vi "SwerveDrive2.0.vi"(6 "Right Trigger":dbl, 8 "RCW":dbl(slide) scale=-1.0..1.0, 9 "STR":dbl(slide) scale=-1.0..1.0, 10 "FWD":dbl(slide) scale=-1.0..1.0, 11 "Gyro":dbl=-0.03423117662966245) -> ()   [LabVIEW 2023]
uses:
  <vilib>/Rock Robotics/WPI/ThirdParty/ADI/ADIS16470/Typedef/ADIS16470 Data.ctl
  <vilib>/Rock Robotics/WPI/ThirdParty/REV Robotics/REVLib/Typedef/Spark MAX Control Type.ctl
  <vilib>/addons/control/pid/NI_PID_pid.lvlib
  <vilib>/addons/control/pid/pid.llb/PID (DBL).vi
panel:
  in  "Do X Pattern":bool=TRUE
  in  "W4 PID":T1={"proportional gain (Kc)"=0.2, "integral time (Ti, min)"=0.0, "derivative time (Td, min)"=0.0}
  in  "W1 PID":T1={"proportional gain (Kc)"=0.2, "integral time (Ti, min)"=0.0, "derivative time (Td, min)"=0.0}
  in  "W2 PID":T1={"proportional gain (Kc)"=0.2, "integral time (Ti, min)"=0.0, "derivative time (Td, min)"=0.0}
  in  "W3 PID":T1={"proportional gain (Kc)"=0.2, "integral time (Ti, min)"=0.0, "derivative time (Td, min)"=0.0}
  out "ADIS16470 Value":T2
  out "W2 Encoder":dbl
  out "W1 Encoder":dbl
  out "WA 4":dbl=135.0
  out "WA 3":dbl=225.0
  out "WA 2":dbl=315.0
  out "WA 1":dbl=45.0
  out "WS 4":dbl
  out "WS 3":dbl
  out "WS 2":dbl
  out "WS 1":dbl
  out "W4 Encoder":dbl
  out "W3 Encoder":dbl
  # "0.2\n0\n0\nfor all"
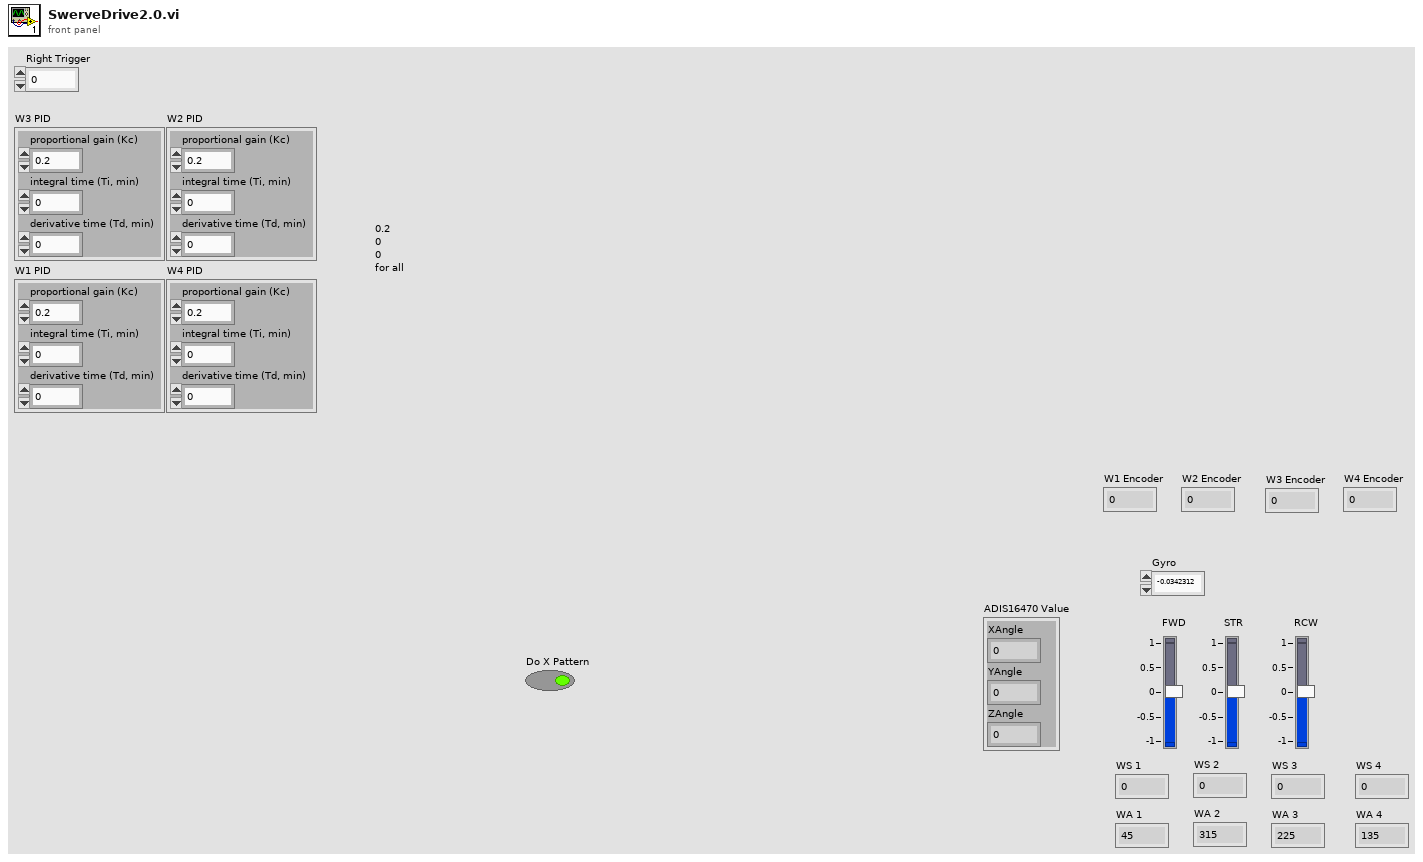
[diagram p1: front panel]
types:
  T1 = cluster{"proportional gain (Kc)":dbl, "integral time (Ti, min)":dbl, "derivative time (Td, min)":dbl}
  T2 = typedef "ADIS16470 Data.ctl" = cluster{"XAngle":dbl, "YAngle":dbl, "ZAngle":dbl}
  T3 = typedef "WPI_JoystickDevRef.ctl" = cluster{"Device":T4}
  T4 = typedef "WPI_JoystickDeviceEnum.ctl" = enum16{"USB 0", "USB 1", "USB 2", "USB 3", "USB 4", "USB 5"}
  T5 = typedef "ADIS16470 Device Reference.ctl" = cluster{"DevStatus":errorcluster, "Hardware Config":T6, "Calibration Complete":refnum<notifier>, "Status Reference":refnum<data-value>, "Data Reference":refnum<data-value>, "Sychronous Process VI":T10, "Cmd FIFO":refnum<k33>, "Source":T11, "Data FIFO":refnum<k33>, "Calibration Time (ms)":u32, "Data Reference":refnum<data-value>}
  T6 = typedef "ADIS16470 Hardware Configuration.ctl" = cluster{"SPI Clock Rate (Hz)":dbl, "IMU SPI Mode (3)":T7, "IMU Reset Pin":T8, "IMU SPI Bus":T9, "IMU Data Ready Pin":T8, "Stall Config":cluster{"Pow2BytesPerRead":u8, "StallTicks":u16, "CsToSclkTicks":u8}}
  T7 = typedef "WPI_SPIMode.ctl" = enum16{"Mode 0 (Clk Idle Low,Sample on Leading)", "Mode 1 (Clk Idle Low,Sample on Trailing)", "Mode 2 (Clk Idle High,Sample on Leading)", "Mode 3 (Clk Idle High,Sample on Trailing)"}
  T8 = typedef "FPGA_DIOChannel.ctl" = enum8{"DIO 0", "DIO 1", "DIO 2", "DIO 3", "DIO 4", "DIO 5", "DIO 6", "DIO 7", "DIO 8", "DIO 9", "DIO MXP 0", "DIO MXP 1", "DIO MXP 2", "DIO MXP 3", "DIO MXP 4", "DIO MXP 5", "DIO MXP 6", "DIO MXP 7", "DIO MXP 8", "DIO MXP 9", "DIO MXP 10", "DIO MXP 11", "DIO MXP 12", "DIO MXP 13", "DIO MXP 14", "DIO MXP 15", "SPI Port CS1", "SPI Port CS2", "SPI Port CS3", "SPI Port MISO", "SPI Port MOSI", "Invalid"}
  T9 = typedef "spi_bus.ctl" = enum16{"SPI On-Board, CS0", "SPI On-Board, CS1", "SPI On-Board, CS2", "SPI On-Board, CS3", "SPI MXP", "Invalid"}
  T10 = typedef "ADIS16470 Process.ctl" = refnum<vi>
  T11 = typedef "FPGA_CounterEncoderSourceConvertionLVSourceType.ctl" = cluster{"DevStatus":errorcluster, "AnalogTriggerMode?":bool, "DigitalMode":cluster{"DIO Channel":T12}, "AnalogTriggerMode":cluster{"AnalogTriggerIndex":T13, "OutputType":T14}}
  T12 = typedef "FPGA_DIODigitalSourceChannel.ctl" = enum8{"DIO 0", "DIO 1", "DIO 2", "DIO 3", "DIO 4", "DIO 5", "DIO 6", "DIO 7", "DIO 8", "DIO 9", "DIO MXP 0", "DIO MXP 1", "DIO MXP 2", "DIO MXP 3", "DIO MXP 4", "DIO MXP 5", "DIO MXP 6", "DIO MXP 7", "DIO MXP 8", "DIO MXP 9", "DIO MXP 10", "DIO MXP 11", "DIO MXP 12", "DIO MXP 13", "DIO MXP 14", "DIO MXP 15", "SPI Port CS1", "SPI Port CS2", "SPI Port CS3", "SPI Port MISO", "SPI Port MOSI", "Disabled"}
  T13 = typedef "FPGA_AnalogTriggerIndex.ctl" = enum8{"Trig 0", "Trig 1", "Trig 2", "Trig 3", "Trig 4", "Trig 5", "Trig 6", "Trig 7", "Invalid"}
  T14 = typedef "FPGA_AnalogTriggerOutType.ctl" = enum16{"InWindow", "TriggerState", "Rising", "Falling"}
  T15 = typedef "WPI_MotorControlDeviceRef.ctl" = cluster{"DeviceStatus":errorcluster, "Type":T16, "PWM":cluster{"PWM Channel":T17, "DeadBand":T18}, "CAN":cluster{"Device Number":u8, "SetOutput VI Ref":variant, "GetOutput VI Ref":variant, "Enable VI Ref":variant, "Disable VI Ref":variant, "Data":variant}, "Invert":bool, "DIO PWM":cluster{"PWM \"Enable\" Channel":T17, "DIOChannel":T8, "PWM Rate":dbl}}
  T16 = typedef "WPI_MotorControlType.ctl" = enum16{"PWM", "CAN", "DIO PWM"}
  T17 = typedef "FPGA_DIOPWMChannel.ctl" = enum8{"PWM 0", "PWM 1", "PWM 2", "PWM 3", "PWM 4", "PWM 5", "PWM 6", "PWM 7", "PWM 8", "PWM 9", "PWM MXP 0", "PWM MXP 1", "PWM MXP 2", "PWM MXP 3", "PWM MXP 4", "PWM MXP 5", "PWM MXP 6", "PWM MXP 7", "PWM MXP 8", "PWM MXP 9", "Invalid"}
  T18 = typedef "WPI_PWMDeadband.ctl" = cluster{"Name":string, "maxPositivePwm":i32, "minPositivePwm":i32, "centerPwm":i32, "maxNegativePwm":i32, "minNegativePwm":i32, "angularRange":u16}
  T19 = typedef "Spark MAX Control Type.ctl" = enum16{"Percent VBus", "Voltage", "Velocity", "Position", "Smart Motion", "Current", "Smart Velocity"}
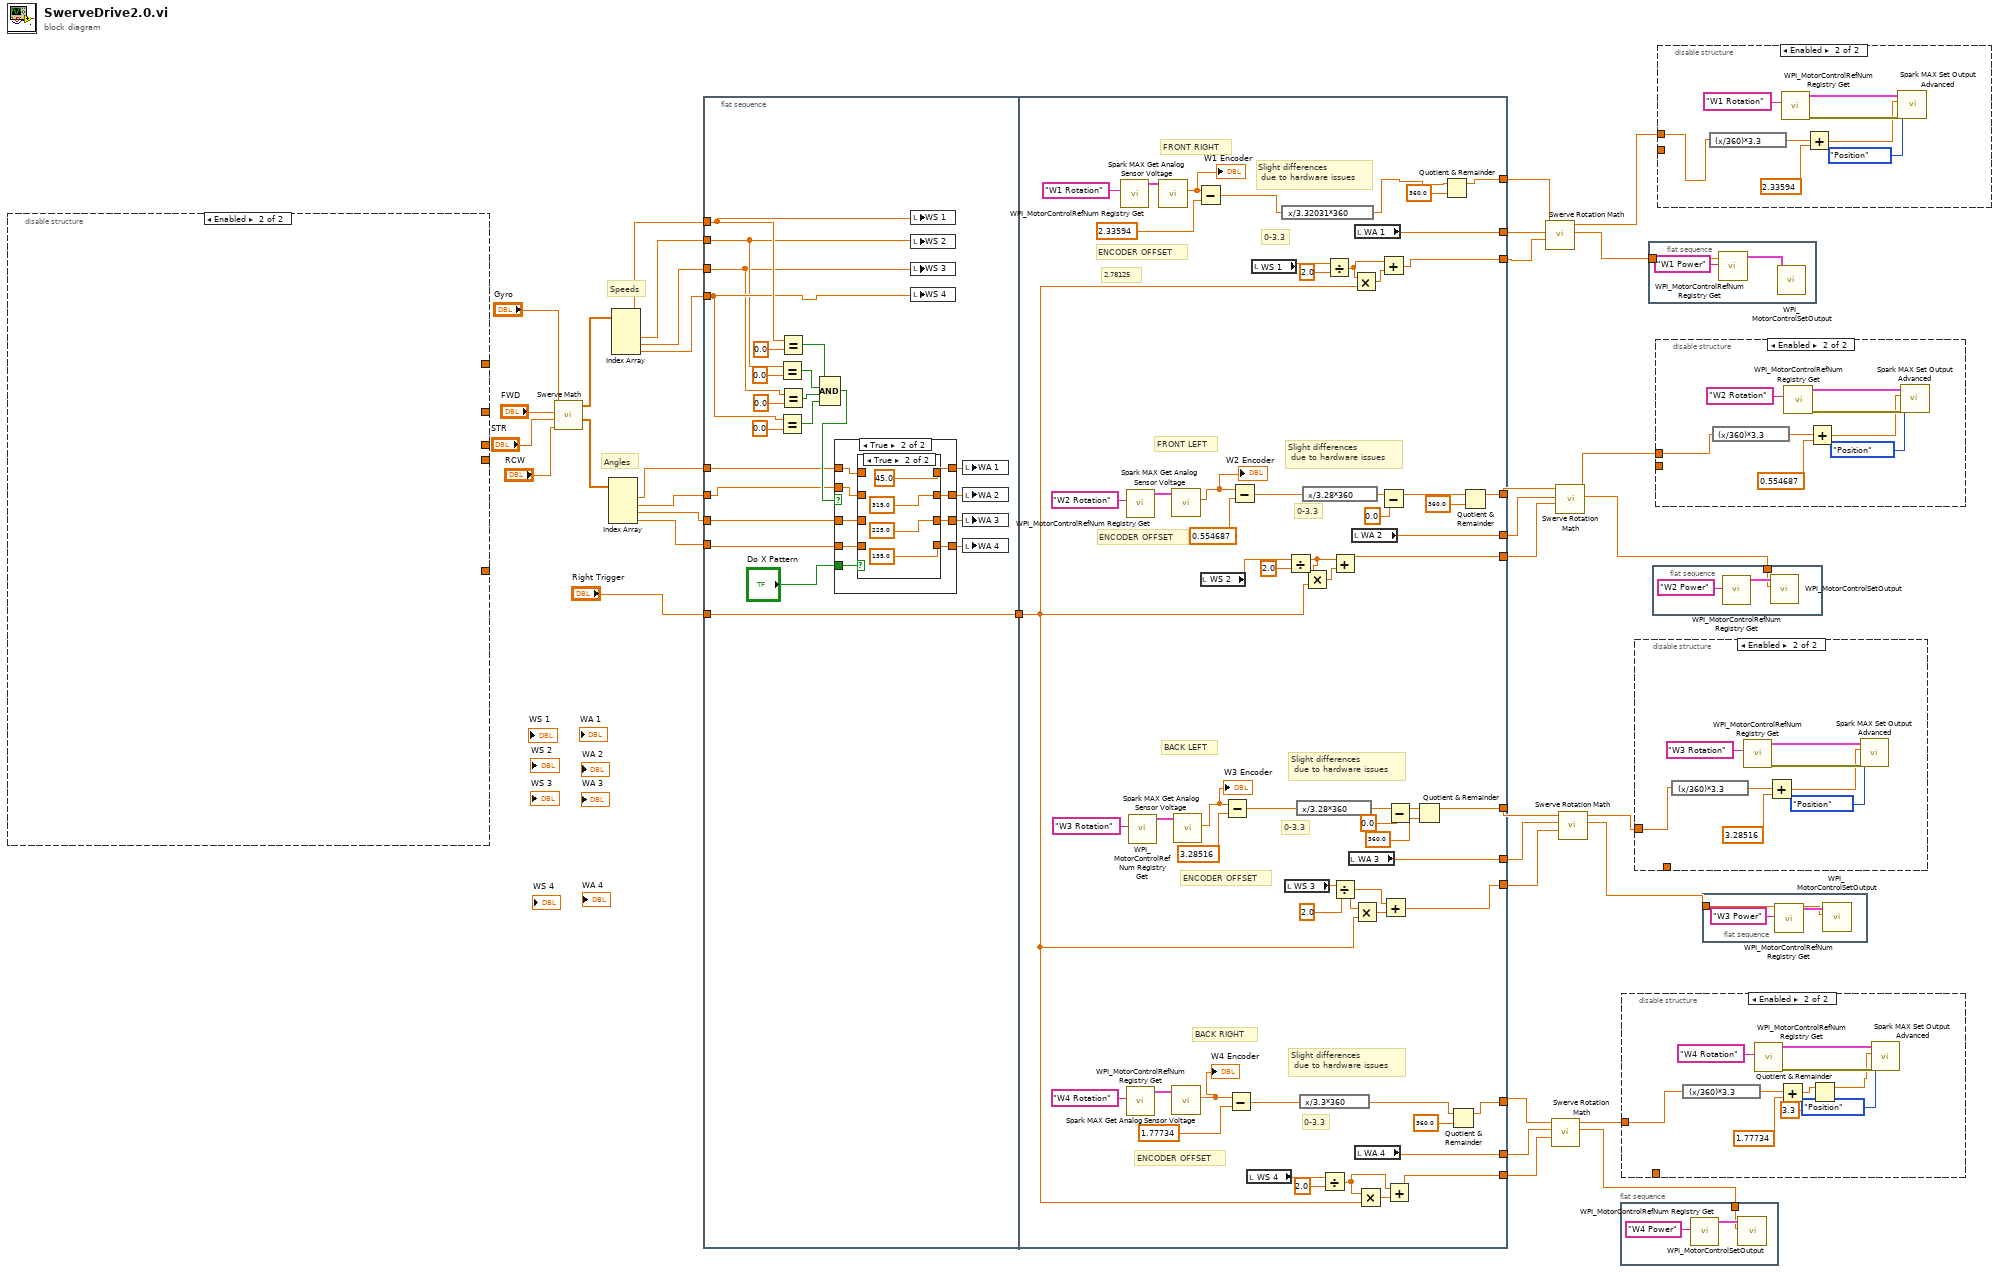
[diagram p0: block diagram]
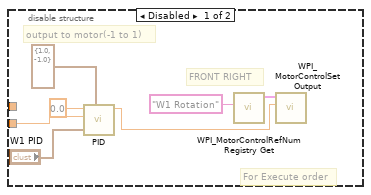
[diagram p2: hidden frame]
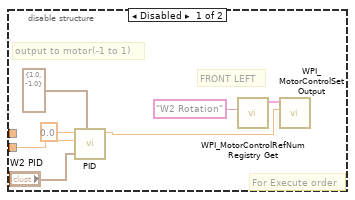
[diagram p3: hidden frame]
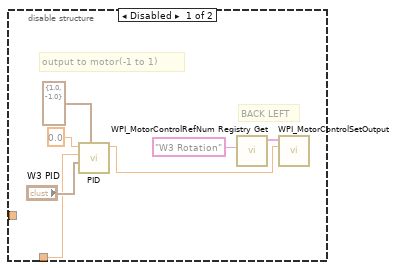
[diagram p4: hidden frame]
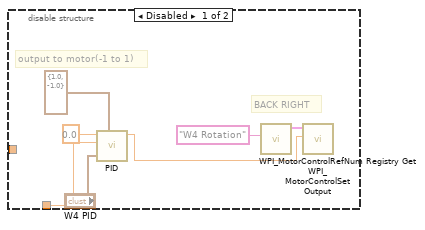
[diagram p5: hidden frame]
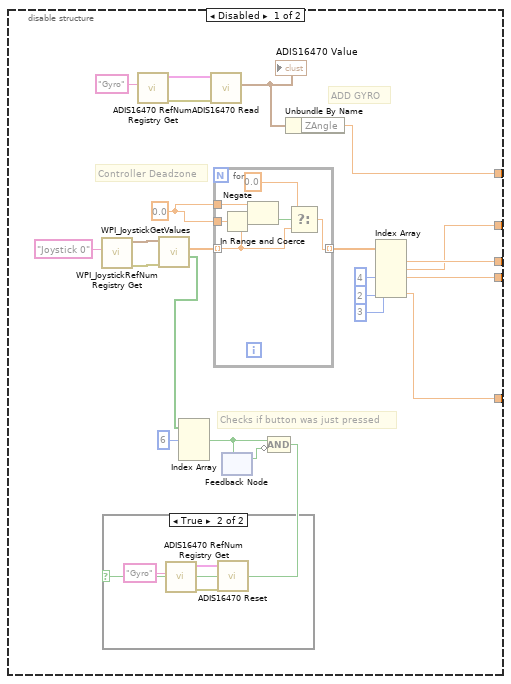
[diagram p6: hidden frame]
diagram:
  # "Angles"
  # "Speeds"
  n1 = disable-structure shown="Enabled" {
    disable-tunnel: [w56 _] -> _
    disable-tunnel: [w55 _] -> _
    disable-tunnel: [w54 _] -> _
    disable-tunnel: [w43 _] -> _
    disable-tunnel: [w40 _] -> _
    frame Disabled {
      w49 = 0.0 ("upper limit")
      # "Checks if button was just pressed"
      # "Controller Deadzone"
      # "ADD GYRO"
      n2 = call <vilib>:"WPI_JoystickRefNum Registry Get.vi"("refnum name"="Joystick 0") -> ("error out"=w59:errorcluster, "JoystickDevRef"=w58:T3)  [unwired: 9 in]
      n3 = call <vilib>:"ADIS16470 RefNum Registry Get.vi"("refnum name"="Gyro") -> ("error out"=w39:errorcluster, "ADIS16470DevRef out"=w37:T5)  [unwired: 9 in]
      n4 = call <vilib>:"WPI_JoystickGetValues.vi"("error in (no error)"=w59, "JoystickDevRef"=w58) -> ("Buttons"=w48:bool[], "Axes"=w51:dbl[])  [unwired: 5 in, 3 out]
      n5 = Index Array(array=w48, index #1=6 ("index")) -> (element #1=w46:bool)  [unwired: 2 in, 2 out]
      n6 = call <vilib>:"ADIS16470 Read.vi"("error in (no error)"=w39, "ADIS16470DevRef"=w37) -> ("ADIS16470 Value"=w52:T2)  [unwired: 6 in, 3 out]
      "ADIS16470 Value" <- w52
      n7 = for {
        tunnel: w51 -> [w64] mode=indexing
        tunnel: [w63] -> w50 mode=indexing
        tunnel: w49 -> [w69]
        tunnel: w49 -> [w68]
        n8 = Negate(x=w68) -> (-x=w67:dbl)
        n9 = In Range and Coerce(upper limit=w69, x=w64, lower limit=w67) -> (In Range?=w66:bool)  [unwired: 1 out]
        n10 = Select(t=0.0, s=w66, f=w64) -> (s? t:f=w63:dbl)
      }
      n11 = feedback #1() -> (w45:bool)  [unwired: 1 in]
      n12 = feedback-in #1(w46) -> ()
      n13 = Compound Arithmetic op=AND(w46, invert w45) -> (w44:bool)
      n14 = case shown="True" w44 {
        frame False {
        }
        frame True {
          n15 = call <vilib>:"ADIS16470 RefNum Registry Get.vi"("refnum name"="Gyro") -> ("error out"=w61:errorcluster, "ADIS16470DevRef out"=w60:T5)  [unwired: 9 in]
          n16 = call <vilib>:"ADIS16470 Reset.vi"("error in (no error)"=w61, "ADIS16470DevRef"=w60) -> ()  [unwired: 8 in, 2 out]
        }
      }
      n17 = Unbundle By Name(w52) -> ("ZAngle"=w43:dbl)
      n18 = Index Array(array=w50, index #3=4 ("index"), index #4=2 ("index"), index #5=3 ("index")) -> (element #1=w56:dbl, element #2=w54:dbl, element #3=w55:dbl, element #5=w40:dbl)  [unwired: 2 in, 1 out]
    }
    frame Enabled {
    }
  }
  n19 = call "Swerve Math.vi"("Gyro"="Gyro", "FWD"="FWD", "STR"="STR", "RCW"="RCW") -> ("Wheel Speeds"=w36:dbl[], "Wheel Angles"=w35:dbl[])  [unwired: 5 in]
  n20 = Index Array(array=w35) -> (element #1=w28:dbl, element #2=w29:dbl, element #3=w30:dbl, element #4=w31:dbl)  [unwired: 4 in]
  n21 = Index Array(array=w36) -> (element #1=w26:dbl, element #2=w24:dbl, element #3=w25:dbl, element #4=w27:dbl)  [unwired: 4 in]
  n22 = flat-sequence {
    tunnel: w31 -> [w73]
    tunnel: w30 -> [w77]
    tunnel: w29 -> [w79]
    tunnel: w28 -> [w81]
    tunnel: w27 -> [w72]
    tunnel: w25 -> [w70]
    tunnel: w26 -> [w83]
    tunnel: w24 -> [w71]
    tunnel: "Right Trigger" -> [w92]
    tunnel: [w92] -> w23
    tunnel: [w174] -> w19
    tunnel: [w173] -> w15
    tunnel: [w123] -> w11
    tunnel: [w172] -> w6
    tunnel: [w124] -> w10
    tunnel: [w132] -> w16
    tunnel: [w130] -> w2
    tunnel: [w147] -> w18
    tunnel: [w151] -> w14
    tunnel: [w143] -> w9
    tunnel: [w141] -> w5
    tunnel: w23 -> [w139]
    tunnel: [w127] -> w7
    frame #0 {
      n23 = Equal?(x=w71, y=0.0) -> (x = y?=w88:bool)
      n24 = Equal?(x=w72, y=0.0) -> (x = y?=w84:bool)
      n25 = Equal?(x=w83, y=0.0) -> (x = y?=w91:bool)
      n26 = Equal?(x=w70, y=0.0) -> (x = y?=w85:bool)
      n27 = Compound Arithmetic op=AND(w91, w88, w85, w84) -> (w82:bool)
      n28 = case shown="True" w82 {
        tunnel: w81 -> [w96 w100]
        tunnel: [w96 w105] -> w80
        tunnel: w79 -> [w95 w99]
        tunnel: [w95 w104] -> w78
        tunnel: w77 -> [w94 w98]
        tunnel: [w94 w103] -> w76
        tunnel: w73 -> [w93 w97]
        tunnel: [w93 w102] -> w75
        tunnel: "Do X Pattern" -> [_ w101]
        frame False {
        }
        frame True {
          n29 = case shown="True" w101 {
            tunnel: [w109 45.0] -> w105
            tunnel: [w108 315.0] -> w104
            tunnel: [w107 225.0] -> w103
            tunnel: [w106 135.0] -> w102
            tunnel: w100 -> [w109 _]
            tunnel: w99 -> [w108 _]
            tunnel: w98 -> [w107 _]
            tunnel: w97 -> [w106 _]
            frame False {
            }
            frame True {
            }
          }
        }
      }
      n30 = local write "WS 1"(w83) -> ()
      n31 = local write "WS 2"(w71) -> ()
      n32 = local write "WS 3"(w70) -> ()
      n33 = local write "WS 4"(w72) -> ()
      n34 = local write "WA 1"(w80) -> ()
      n35 = local write "WA 2"(w78) -> ()
      n36 = local write "WA 3"(w76) -> ()
      n37 = local write "WA 4"(w75) -> ()
    }
    frame #1 {
      # "2.78125"
      # "Slight differences\n due to hardware issues"
      # "Slight differences\n due to hardware issues"
      # "Slight differences\n due to hardware issues"
      # "Slight differences\n due to hardware issues"
      # "BACK RIGHT"
      # "BACK LEFT"
      # "FRONT LEFT"
      # "FRONT RIGHT"
      # "ENCODER OFFSET"
      # "ENCODER OFFSET"
      # "ENCODER OFFSET"
      # "ENCODER OFFSET"
      # "0-3.3"
      # "0-3.3"
      # "0-3.3"
      # "0-3.3"
      n38 = call <vilib>:"WPI_MotorControlRefNum Registry Get.vi"("refnum name"="W1 Rotation") -> ("MotorControlDevRef"=w171:T15)  [unwired: 9 in, 1 out]
      n39 = call <vilib>:"WPI_MotorControlRefNum Registry Get.vi"("refnum name"="W2 Rotation") -> ("MotorControlDevRef"=w160:T15)  [unwired: 9 in, 1 out]
      n40 = call <vilib>:"WPI_MotorControlRefNum Registry Get.vi"("refnum name"="W4 Rotation") -> ("MotorControlDevRef"=w166:T15)  [unwired: 9 in, 1 out]
      n41 = call <vilib>:"WPI_MotorControlRefNum Registry Get.vi"("refnum name"="W3 Rotation") -> ("MotorControlDevRef"=w168:T15)  [unwired: 9 in, 1 out]
      n42 = call <vilib>:"Spark MAX Get Analog Sensor Voltage.vi"("MotorControlDevRef in"=w171) -> ("Analog Sensor Voltage"=w119:dbl)  [unwired: 7 in, 3 out]
      "W1 Encoder" <- w119
      n43 = call <vilib>:"Spark MAX Get Analog Sensor Voltage.vi"("MotorControlDevRef in"=w160) -> ("Analog Sensor Voltage"=w121:dbl)  [unwired: 7 in, 3 out]
      "W2 Encoder" <- w121
      n44 = call <vilib>:"Spark MAX Get Analog Sensor Voltage.vi"("MotorControlDevRef in"=w166) -> ("Analog Sensor Voltage"=w115:dbl)  [unwired: 7 in, 3 out]
      "W4 Encoder" <- w115
      n45 = call <vilib>:"Spark MAX Get Analog Sensor Voltage.vi"("MotorControlDevRef in"=w168) -> ("Analog Sensor Voltage"=w117:dbl)  [unwired: 7 in, 3 out]
      "W3 Encoder" <- w117
      n46 = Subtract(x=w119, y=2.33594) -> (x-y=w118:dbl)
      n47 = local read "WS 2"() -> (w163:dbl)
      n48 = Subtract(x=w117, y=3.28516) -> (x-y=w116:dbl)
      n49 = Subtract(x=w115, y=1.77734 ("x")) -> (x-y=w114:dbl)
      n50 = Subtract(x=w121, y=0.554687) -> (x-y=w120:dbl)
      n51 = local read "WS 4"() -> (w161:dbl)
      n52 = local read "WS 1"() -> (w164:dbl)
      n53 = expression code="x/3.32031*360"(w118) -> (w122:dbl)
      n54 = local read "WS 3"() -> (w162:dbl)
      n55 = Divide(x=w163, y=2.0) -> (x/y=w149:dbl)
      n56 = expression code="x/3.28*360"(w116) -> (w138:dbl)
      n57 = expression code="x/3.3*360"(w114) -> (w128:dbl)
      n58 = expression code="x/3.28*360"(w120) -> (w134:dbl)
      n59 = Multiply(x=w149, y=w139) -> (x*y=w150:dbl)
      n60 = Divide(x=w161, y=2.0) -> (x/y=w140:dbl)
      n61 = Divide(x=w164, y=2.0) -> (x/y=w146:dbl)
      n62 = Add(x=w149, y=w150) -> (x+y=w151:dbl)
      n63 = Divide(x=w162, y=2.0) -> (x/y=w144:dbl)
      n64 = local read "WA 3"() -> (w123:dbl)
      n65 = Multiply(x=w146, y=w139) -> (x*y=w148:dbl)
      n66 = local read "WA 2"() -> (w173:dbl)
      n67 = Multiply(x=w144, y=w139) -> (x*y=w145:dbl)
      n68 = local read "WA 1"() -> (w174:dbl)
      n69 = local read "WA 4"() -> (w172:dbl)
      n70 = Multiply(x=w140, y=w139) -> (x*y=w142:dbl)
      n71 = Add(x=w146, y=w148) -> (x+y=w147:dbl)
      n72 = Subtract(x=w134, y=0.0) -> (x-y=w126:dbl)
      n73 = Add(x=w144, y=w145) -> (x+y=w143:dbl)
      n74 = Add(x=w140, y=w142) -> (x+y=w141:dbl)
      n75 = Subtract(x=w138, y=0.0) -> (x-y=w137:dbl)
      n76 = Quotient & Remainder(x=w137, y=360.0) -> (x-y*floor(x/y)=w124:dbl)  [unwired: 1 out]
      n77 = Quotient & Remainder(x=w122, y=360.0) -> (x-y*floor(x/y)=w130:dbl)  [unwired: 1 out]
      n78 = Quotient & Remainder(x=w128, y=360.0) -> (x-y*floor(x/y)=w127:dbl)  [unwired: 1 out]
      n79 = Quotient & Remainder(x=w126, y=360.0) -> (x-y*floor(x/y)=w132:dbl)  [unwired: 1 out]
    }
  }
  n80 = call "Swerve Rotation Math.vi"("Wheel Speed"=w18, "Wheel Angle"=w19, "Encoder"=w2) -> ("Wheel Speed"=w20:dbl, "Goal"=w21:dbl)  [unwired: 7 in]
  n81 = call "Swerve Rotation Math.vi"("Wheel Speed"=w5, "Wheel Angle"=w6, "Encoder"=w7) -> ("Wheel Speed"=w4:dbl, "Goal"=w3:dbl)  [unwired: 7 in]
  n82 = call "Swerve Rotation Math.vi"("Wheel Speed"=w14, "Wheel Angle"=w15, "Encoder"=w16) -> ("Wheel Speed"=w13:dbl, "Goal"=w17:dbl)  [unwired: 7 in]
  n83 = call "Swerve Rotation Math.vi"("Wheel Speed"=w9, "Wheel Angle"=w11, "Encoder"=w10) -> ("Wheel Speed"=w8:dbl, "Goal"=w12:dbl)  [unwired: 7 in]
  n84 = flat-sequence {
    tunnel: w4 -> [w175]
    frame #0 {
      n85 = call <vilib>:"WPI_MotorControlRefNum Registry Get.vi"("refnum name"="W4 Power") -> ("MotorControlDevRef"=w176:T15)  [unwired: 9 in, 1 out]
      n86 = call <vilib>:"WPI_MotorControlSetOutput.vi"("Output"=w175, "MotorControlDevRef"=w176) -> ()  [unwired: 7 in, 3 out]
    }
  }
  n87 = disable-structure shown="Enabled" {
    disable-tunnel: _ -> [w185 _]
    disable-tunnel: w3 -> [_ w189]
    frame Disabled {
      # "output to motor(-1 to 1)"
      # "BACK RIGHT"
      n88 = call-poly <vilib>:"PID.vi"("output range"=cluster{"output high":dbl, "output low":dbl} {"output high"=1.0, "output low"=-1.0}, "PID gains"="W4 PID", "process variable"=w185, "setpoint"=0.0) -> ("output"=w183:dbl)  [unwired: 6 in, 1 out]
      n89 = call <vilib>:"WPI_MotorControlRefNum Registry Get.vi"("refnum name"="W4 Rotation") -> ("MotorControlDevRef"=w184:T15)  [unwired: 9 in, 1 out]
      n90 = call <vilib>:"WPI_MotorControlSetOutput.vi"("Output"=w183, "MotorControlDevRef"=w184) -> ("Motor Output"=w181:dbl)  [unwired: 7 in, 2 out]
    }
    frame Enabled {
      n91 = expression code="(x/360)*3.3"(w189) -> (w190:dbl)
      n92 = call <vilib>:"WPI_MotorControlRefNum Registry Get.vi"("refnum name"="W4 Rotation") -> ("error out"=w192:errorcluster, "MotorControlDevRef"=w193:T15)  [unwired: 9 in]
      n93 = Add(x=w190, y=1.77734) -> (x+y=w188:dbl)
      n94 = Quotient & Remainder(x=w188, y=3.3) -> (x-y*floor(x/y)=w186:dbl)  [unwired: 1 out]
      n95 = call <vilib>:"Spark MAX Set Output Advanced.vi"("error in (no error)"=w192, "Control Mode"=Spark_MAX_Control_Type."Position", "Setpoint"=w186, "MotorControlDevRef"=w193) -> ()  [unwired: 6 in, 2 out]
    }
  }
  n96 = disable-structure shown="Enabled" {
    disable-tunnel: _ -> [w199 _]
    disable-tunnel: w12 -> [_ w203]
    frame Disabled {
      # "BACK LEFT"
      # "output to motor(-1 to 1)"
      n97 = call-poly <vilib>:"PID.vi"("output range"=cluster{"output high":dbl, "output low":dbl} {"output high"=1.0, "output low"=-1.0}, "PID gains"="W3 PID", "process variable"=w199, "setpoint"=0.0) -> ("output"=w197:dbl)  [unwired: 6 in, 1 out]
      n98 = call <vilib>:"WPI_MotorControlRefNum Registry Get.vi"("refnum name"="W3 Rotation") -> ("MotorControlDevRef"=w198:T15)  [unwired: 9 in, 1 out]
      n99 = call <vilib>:"WPI_MotorControlSetOutput.vi"("Output"=w197, "MotorControlDevRef"=w198) -> ()  [unwired: 7 in, 3 out]
    }
    frame Enabled {
      n100 = expression code="(x/360)*3.3"(w203) -> (w205:dbl)
      n101 = call <vilib>:"WPI_MotorControlRefNum Registry Get.vi"("refnum name"="W3 Rotation") -> ("error out"=w207:errorcluster, "MotorControlDevRef"=w208:T15)  [unwired: 9 in]
      n102 = Add(x=w205, y=3.28516) -> (x+y=w204:dbl)
      n103 = call <vilib>:"Spark MAX Set Output Advanced.vi"("error in (no error)"=w207, "Control Mode"=Spark_MAX_Control_Type."Position", "Setpoint"=w204, "MotorControlDevRef"=w208) -> ()  [unwired: 6 in, 2 out]
    }
  }
  n104 = flat-sequence {
    tunnel: w20 -> [w211]
    frame #0 {
      n105 = call <vilib>:"WPI_MotorControlRefNum Registry Get.vi"("refnum name"="W1 Power") -> ("MotorControlDevRef"=w212:T15)  [unwired: 9 in, 1 out]
      n106 = call <vilib>:"WPI_MotorControlSetOutput.vi"("Output"=w211, "MotorControlDevRef"=w212) -> ()  [unwired: 7 in, 3 out]
    }
  }
  n107 = flat-sequence {
    tunnel: w13 -> [w214]
    frame #0 {
      n108 = call <vilib>:"WPI_MotorControlRefNum Registry Get.vi"("refnum name"="W2 Power") -> ("MotorControlDevRef"=w215:T15)  [unwired: 9 in, 1 out]
      n109 = call <vilib>:"WPI_MotorControlSetOutput.vi"("Output"=w214, "MotorControlDevRef"=w215) -> ()  [unwired: 7 in, 3 out]
    }
  }
  n110 = disable-structure shown="Enabled" {
    disable-tunnel: _ -> [w221 _]
    disable-tunnel: w17 -> [_ w225]
    frame Disabled {
      # "FRONT LEFT"
      # "output to motor(-1 to 1)"
      # "For Execute order"
      n111 = call-poly <vilib>:"PID.vi"("output range"=cluster{"output high":dbl, "output low":dbl} {"output high"=1.0, "output low"=-1.0}, "PID gains"="W2 PID", "process variable"=w221, "setpoint"=0.0) -> ("output"=w219:dbl)  [unwired: 6 in, 1 out]
      n112 = call <vilib>:"WPI_MotorControlRefNum Registry Get.vi"("refnum name"="W2 Rotation") -> ("MotorControlDevRef"=w220:T15)  [unwired: 9 in, 1 out]
      n113 = call <vilib>:"WPI_MotorControlSetOutput.vi"("Output"=w219, "MotorControlDevRef"=w220) -> ("Motor Output"=w217:dbl)  [unwired: 7 in, 2 out]
    }
    frame Enabled {
      n114 = expression code="(x/360)*3.3"(w225) -> (w227:dbl)
      n115 = call <vilib>:"WPI_MotorControlRefNum Registry Get.vi"("refnum name"="W2 Rotation") -> ("error out"=w229:errorcluster, "MotorControlDevRef"=w230:T15)  [unwired: 9 in]
      n116 = Add(x=w227, y=0.554687) -> (x+y=w226:dbl)
      n117 = call <vilib>:"Spark MAX Set Output Advanced.vi"("error in (no error)"=w229, "Control Mode"=Spark_MAX_Control_Type."Position", "Setpoint"=w226, "MotorControlDevRef"=w230) -> ()  [unwired: 6 in, 2 out]
    }
  }
  n118 = disable-structure shown="Enabled" {
    disable-tunnel: _ -> [w237 _]
    disable-tunnel: w21 -> [_ w241]
    frame Disabled {
      # "FRONT RIGHT"
      # "output to motor(-1 to 1)"
      # "For Execute order"
      n119 = call-poly <vilib>:"PID.vi"("output range"=cluster{"output high":dbl, "output low":dbl} {"output high"=1.0, "output low"=-1.0}, "PID gains"="W1 PID", "process variable"=w237, "setpoint"=0.0) -> ("output"=w235:dbl)  [unwired: 6 in, 1 out]
      n120 = call <vilib>:"WPI_MotorControlRefNum Registry Get.vi"("refnum name"="W1 Rotation") -> ("MotorControlDevRef"=w236:T15)  [unwired: 9 in, 1 out]
      n121 = call <vilib>:"WPI_MotorControlSetOutput.vi"("Output"=w235, "MotorControlDevRef"=w236) -> ("Motor Output"=w233:dbl)  [unwired: 7 in, 2 out]
    }
    frame Enabled {
      n122 = expression code="(x/360)*3.3"(w241) -> (w243:dbl)
      n123 = call <vilib>:"WPI_MotorControlRefNum Registry Get.vi"("refnum name"="W1 Rotation") -> ("error out"=w245:errorcluster, "MotorControlDevRef"=w246:T15)  [unwired: 9 in]
      n124 = Add(x=w243, y=2.33594) -> (x+y=w242:dbl)
      n125 = call <vilib>:"Spark MAX Set Output Advanced.vi"("error in (no error)"=w245, "Control Mode"=Spark_MAX_Control_Type."Position", "Setpoint"=w242, "MotorControlDevRef"=w246) -> ()  [unwired: 6 in, 2 out]
    }
  }
  n126 = flat-sequence {
    tunnel: w8 -> [w249]
    frame #0 {
      n127 = call <vilib>:"WPI_MotorControlRefNum Registry Get.vi"("refnum name"="W3 Power") -> ("MotorControlDevRef"=w250:T15)  [unwired: 9 in, 1 out]
      n128 = call <vilib>:"WPI_MotorControlSetOutput.vi"("Output"=w249, "MotorControlDevRef"=w250) -> ()  [unwired: 7 in, 3 out]
    }
  }
